vi "Validate.vi"(8 "error in (no error)":errorcluster, 11 "Build in":refnum<class "AB_Build.lvclass">) -> (0 "error out":errorcluster, 3 "Build out":refnum<class "AB_Build.lvclass">)   [LabVIEW 2020, in "AB_Build.lvclass"]
uses:
  <vilib>/AppBuilder/AB_Classes/Build/AB_Build.lvclass
  <resource>/Framework/Providers/Common/provcom_StringGlobals.vi
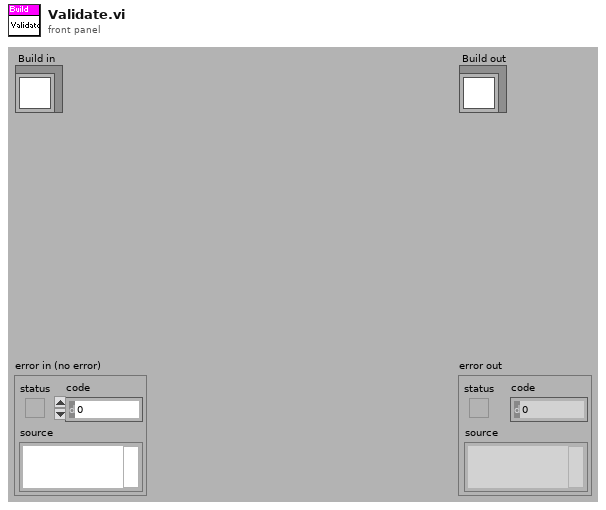
[diagram p1: front panel]
types:
  T1 = typedef "AB_Source_Inclusion.ctl" = enum16{"IncludeIfReferenced", "Include", "Exclude", "TopLevel"}
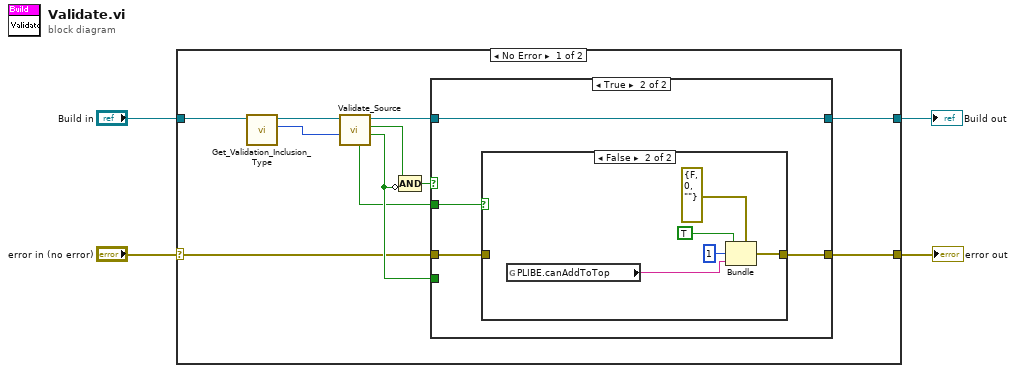
[diagram p0: block diagram]
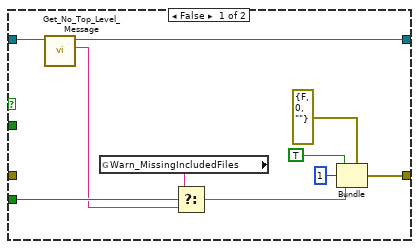
[diagram p2: hidden frame]
diagram:
  n1 = case shown="No Error" "error in (no error)" {
    selector: "error in (no error)" -> [w11 w37]
    tunnel: [w12 w37] -> w3
    tunnel: [w9 w36] -> w1
    tunnel: "Build in" -> [w8 w36]
    frame No Error {
      n2 = call-dynamic "Get_Validation_Inclusion_Type.vi"("AB_Build in"=w8) -> ("sourceInclusion"=w6:T1, "AB_Build out"=w7:refnum<class "AB_Build.lvclass">)  [unwired: 8 in, 1 out]
      n3 = call-dynamic "Validate_Source.vi"("sourceInclusion"=w6, "AB_Build in"=w7) -> ("missingFiles"=w13:bool, "includedFiles"=w14:bool, "AB_Build out"=w10:refnum<class "AB_Build.lvclass">, "canAddToTop"=w5:bool)  [unwired: 5 in, 1 out]
      n4 = Compound Arithmetic op=AND(w14, invert w13) -> (w15:bool)
      n5 = case shown="True" w15 {
        tunnel: [w22 w28] -> w12
        tunnel: w11 -> [_ w26]
        tunnel: w13 -> [w21 _]
        tunnel: w10 -> [w18 w29]
        tunnel: [w17 w29] -> w9
        tunnel: w5 -> [_ w27]
        frame False {
          n6 = call-dynamic "Get_No_Top_Level_Message.vi"("Build in"=w18) -> ("No top level VI"=w16:string, "Build out"=w17:refnum<class "AB_Build.lvclass">)  [unwired: 9 in]
          n7 = global read "provcom_StringGlobals.vi" "Warn_MissingIncludedFiles"() -> (w20:string)
          n8 = Select(t=w20, s=w21, f=w16) -> (s? t:f=w19:string)
          n9 = Bundle(cluster=errorcluster {"status"=FALSE, "code"=0, "source"=""} ("error IO"), "status"=TRUE, "code"=1, "source"=w19) -> (w22:errorcluster)
        }
        frame True {
          n10 = case shown="False" w27 {
            tunnel: [w30 w31] -> w28
            tunnel: w26 -> [w30 _]
            frame True {
            }
            frame False {
              n11 = global read "provcom_StringGlobals.vi" "PLIBE.canAddToTop"() -> (w32:string)
              n12 = Bundle(cluster=errorcluster {"status"=FALSE, "code"=0, "source"=""} ("error IO"), "status"=TRUE, "code"=1, "source"=w32) -> (w31:errorcluster)
            }
          }
        }
      }
    }
    frame Error {
    }
  }
  "error out" <- w3
  "Build out" <- w1
